vi "Filter Item.vi"(6 "Case Sensitive?":bool, 7 "Filter Type":T1, 8 "error in (no error)":errorcluster, 9 "Filter Value":string, 10 "Filter Column":T2, 11 "Control in":refnum<class "Control.lvclass">) -> (0 "error out":errorcluster, 2 "Include?":bool, 3 "Control out":refnum<class "Control.lvclass">)   [LabVIEW 2020, in "VI Properties Editor.lvlib" / "Control.lvclass"]
doc: "Checks whether <B>Item in</B> will be included in a filter defined by the other inputs."
uses:
  Control.lvclass
  CTLs/Filter Column.ctl
  CTLs/Filter Type.ctl
  VI Properties Editor.lvlib
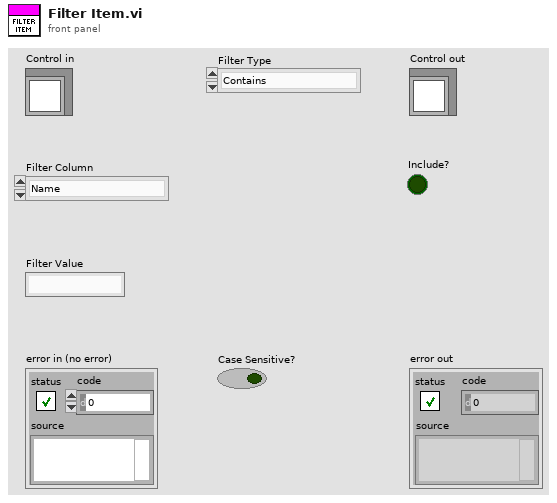
[diagram p1: front panel]
types:
  T1 = typedef "VI Properties Editor.lvlib/Filter Type.ctl" = enum16{"Contains", "Equals", "Starts with", "Ends with", "Is empty", "Does not contain", "Does not equal", "Is not empty"}
  T2 = typedef "VI Properties Editor.lvlib/Filter Column.ctl" = enum16{"Name", "Path", "Type", "Window Title", "Description", "Help Path", "Help Tag", "Custom Title?", "Reentrancy", "Inlined?", "Help URL", "Help Type", "Allow Debugging?", "Auto Error Handling?", "Run When Opened?", "Suspend When Called?", "Priority", "Preferred Exec Sytem", "Control Label", "Control Caption", "Control Description", "Control Tip Strip"}
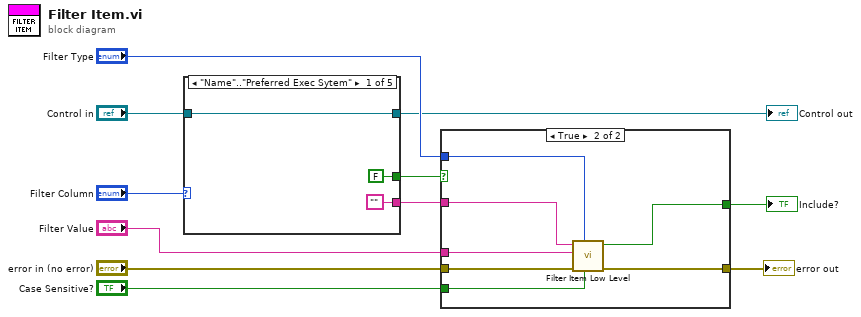
[diagram p0: block diagram]
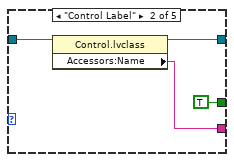
[diagram p2: hidden frame]
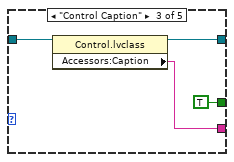
[diagram p3: hidden frame]
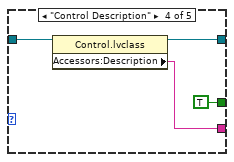
[diagram p4: hidden frame]
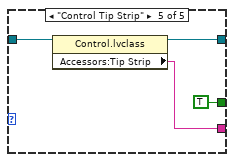
[diagram p5: hidden frame]
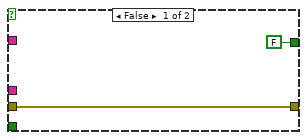
[diagram p6: hidden frame]
diagram:
  n1 = case shown="\"Name\"..\"Preferred Exec Sytem\"" "Filter Column" {
    tunnel: ["" w16 w20 w24 w28] -> w11
    tunnel: "Control in" -> [w14 w18 w22 w26 w30]
    tunnel: [w14 w17 w21 w25 w29] -> w6
    tunnel: [FALSE TRUE TRUE TRUE TRUE] -> w2
    frame "Name".."Preferred Exec Sytem" {
    }
    frame "Control Label" {
      n2 = property class="Control.lvclass"(reference=w18) -> (reference out=w17:refnum<class "Control.lvclass">, "Accessors:Name"=w16:string)  [unwired: 1 in, 1 out]
    }
    frame "Control Caption" {
      n3 = property class="Control.lvclass"(reference=w22) -> (reference out=w21:refnum<class "Control.lvclass">, "Accessors:Caption"=w20:string)  [unwired: 1 in, 1 out]
    }
    frame "Control Description" {
      n4 = property class="Control.lvclass"(reference=w26) -> (reference out=w25:refnum<class "Control.lvclass">, "Accessors:Description"=w24:string)  [unwired: 1 in, 1 out]
    }
    frame "Control Tip Strip" {
      n5 = property class="Control.lvclass"(reference=w30) -> (reference out=w29:refnum<class "Control.lvclass">, "Accessors:Tip Strip"=w28:string)  [unwired: 1 in, 1 out]
    }
  }
  "Control out" <- w6
  n6 = case shown="True" w2 {
    tunnel: w11 -> [_ w39]
    tunnel: "Filter Type" -> [_ w38]
    tunnel: "error in (no error)" -> [w31 w37]
    tunnel: [w31 w36] -> w5
    tunnel: [FALSE ("Include?") w35] -> w4
    tunnel: "Filter Value" -> [_ w34]
    tunnel: "Case Sensitive?" -> [_ w33]
    frame False {
    }
    frame True {
      n7 = call "Filter Item Low Level.vi"("Case Sensitive?"=w33, "Filter Type"=w38, "error in (no error)"=w37, "Filter Value"=w34, "Item Value"=w39) -> ("error out"=w36:errorcluster, "Include?"=w35:bool)  [unwired: 5 in]
    }
  }
  "error out" <- w5
  "Include?" <- w4
